vi "G4BaseTemplate_Singleton_5x6x5_ReadWriteAttributeWithRef.vi"(0 "reference in":refnum<class "G4BaseTemplate_Singleton_5x6x5.lvclass">, 11 "Error In":errorcluster) -> (4 "reference out":refnum<class "G4BaseTemplate_Singleton_5x6x5.lvclass">, 15 "Error Out":errorcluster)   [LabVIEW 2020]
uses:
  <resource>/Framework/Providers/Open_GDS/ClassProviders/Provider_EndevoGOOP400/Templates/G4BaseTemplate_Singleton_5x6x5/G4BaseTemplate_Singleton_5x6x5.lvclass
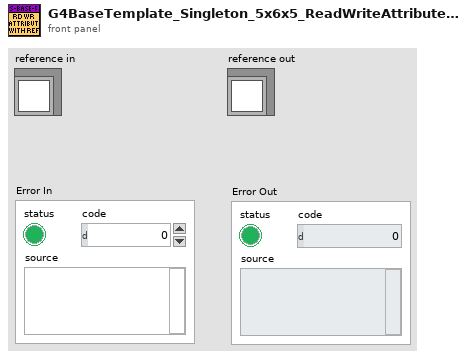
[diagram p1: front panel]
types:
  T1 = typedef "G4BaseTemplate_Singleton_5x6x5.lvclass/ObjectAttributes.ctl" = cluster{"Attribute1":dbl}
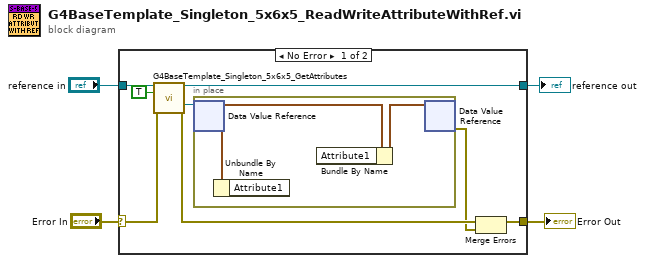
[diagram p0: block diagram]
diagram:
  n1 = case shown="No Error" "Error In" {
    selector: "Error In" -> [w11 w16]
    tunnel: [w12 w16] -> w3
    tunnel: "reference in" -> [w7 w15]
    tunnel: [w6 w15] -> w1
    frame No Error {
      n2 = call <resource>:"G4BaseTemplate_Singleton_5x6x5_GetAttributes.vi"("reference in"=w7, "OnlyGetDvrReference(False)"=TRUE, "Error In"=w11) -> ("reference out"=w6:refnum<class "G4BaseTemplate_Singleton_5x6x5.lvclass">, "DataRef"=w10:refnum<data-value>, "Error Out"=w9:errorcluster)  [unwired: 9 in, 1 out]
      n3 = in-place {
        n4 = in-place-dvr #1(w10) -> (w13:T1)  [unwired: 1 out]
        n5 = Unbundle By Name(w13) -> ()  [unwired: 1 out]
        n6 = Bundle By Name(cluster=w13) -> (w14:T1)  [unwired: 1 in]
        n7 = in-place-dvr #1(w14) -> (w8:errorcluster)  [unwired: 1 out]
      }
      n8 = Merge Errors(w9, w8) -> (w12:errorcluster)
    }
    frame Error {
    }
  }
  "Error Out" <- w3
  "reference out" <- w1
